vi "Read from Hardware.vi"(8 "error in":errorcluster, 10 "Values in":dbl[](array[numeric]), 11 "Tx Execution Unit Implementation in":refnum<class "Tx Generic Execution Unit.lvclass">) -> (0 "error out":errorcluster, 2 "Values out":dbl[](array[numeric]), 3 "Tx Execution Unit Implementation out":refnum<class "Tx Generic Execution Unit.lvclass">)   [LabVIEW 2025, in "AIM ARINC 664 Engine.lvlib" / "Implementation.lvlib" / "Tx Generic Execution Unit.lvclass"]
uses:
  Tx Generic Execution Unit.lvclass
  Tx Generic Execution Unit.lvclass/Tx Generic Execution Unit.ctl
  <instrlib>/AIM GmbH/_AIM 664/AIM664LV.lvlib
  <vilib>/Utility/SystemLogging/NI_SystemLogging.lvlib
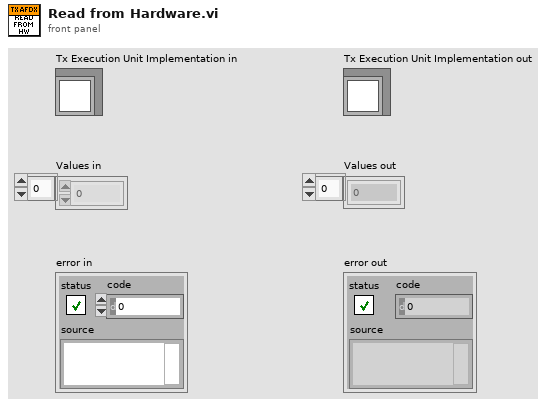
[diagram p1: front panel]
types:
  T1 = cluster{"QueueStatus":i32, "BytesReloadable":u32, "FramesSent":u32, "FramesInCycQueue":u32}
  T2 = cluster{"TxStatus":u32, "Frames":u32, "TransmitMode":u32, "FramesPortB":u32}
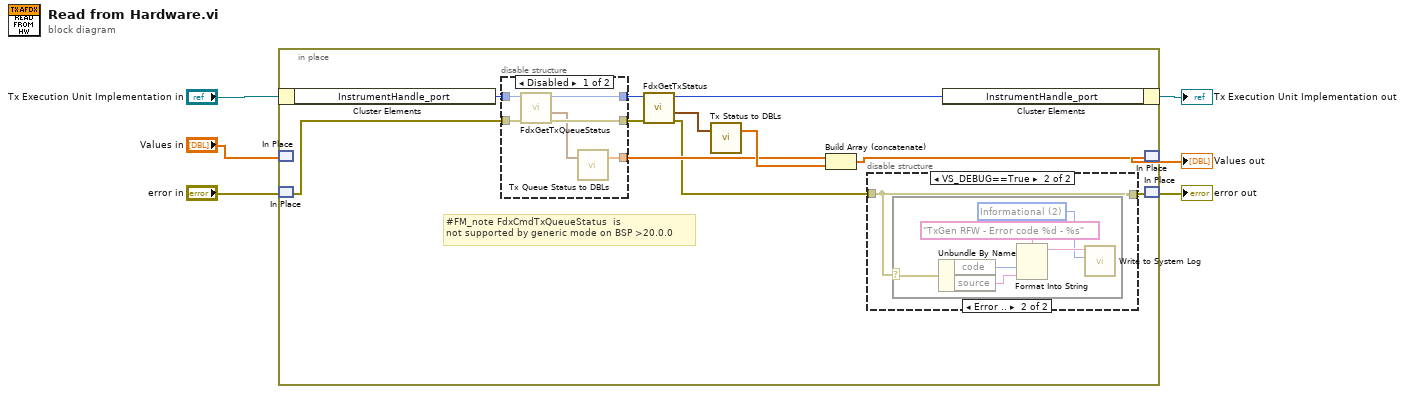
[diagram p0: block diagram]
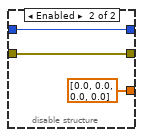
[diagram p2: hidden frame]
diagram:
  n1 = in-place {
    # "#FM_note FdxCmdTxQueueStatus  is \nnot supported by generic mode on BSP >20.0.0"
    n2 = in-place-cluster #1("Tx Execution Unit Implementation in") -> ("InstrumentHandle_port"=w16:u32)
    n3 = in-place-match #2("Values in") -> ()  [unwired: 1 out]
    n4 = in-place-match #3("error in") -> (w14:errorcluster)
    n5 = disable-structure shown="Disabled" {
      disable-tunnel: [w23 w26] -> w17
      disable-tunnel: w16 -> [w22 w25]
      disable-tunnel: [w21 w25] -> w15
      disable-tunnel: w14 -> [w20 w26]
      disable-tunnel: [w18 dbl[] [0.0, 0.0, 0.0, 0.0] ("TxQueueStatusDBLs")] -> w10
      frame Disabled {
        n6 = call <instrlib>:"FdxGetTxQueueStatus.vi"("error in"=w20, "InstrumentHandle"=w22) -> ("error out"=w23:errorcluster, "TxQueueStatus"=w19:T1, "InstrumentHandle"=w21:u32)  [unwired: 7 in]
        n7 = call "Tx Queue Status to DBLs.vi"("TxQueueStatus"=w19) -> ("TxQueueStatusDBLs"=w18:dbl[])  [unwired: 2 in]
      }
      frame Enabled {
      }
    }
    n8 = call <instrlib>:"FdxGetTxStatus.vi"("error in"=w17, "InstrumentHandle_port"=w15) -> ("error out"=w8:errorcluster, "TxStatus"=w12:T2, "InstrumentHandle_port"=w13:u32)  [unwired: 7 in]
    n9 = call "Tx Status to DBLs.vi"("TxStatus"=w12) -> ("TxStatusDBLs"=w11:dbl[])  [unwired: 2 in]
    n10 = Build Array (concatenate)(w10, w11) -> (w9:dbl[])
    n11 = disable-structure shown="VS_DEBUG==True" {
      disable-tunnel: w8 -> [w27 w28]
      disable-tunnel: [w27 w28] -> w7
      frame condition #0 (active) {
      }
      frame condition #1 {
        n12 = case shown="Error .." w28 {
          selector: w28 -> [_ w29]
          frame No Error {
          }
          frame Error {
            w32 = 2 items=["Error", "Warning", "Informational"] ("severity")
            n13 = Unbundle By Name(w29) -> ("code"=w31:i32, "source"=w30:string)
            n14 = Format Into String(format string="TxGen RFW - Error code %d - %s", w31, w30) -> (resulting string=w33:string)  [unwired: 2 in, 1 out]
            n15 = call <vilib>:"Write to System Log.vi"("severity"=w32, "message"=w33) -> ()  [unwired: 9 in, 1 out]
          }
        }
      }
    }
    n16 = in-place-cluster #1("InstrumentHandle_port"=w13) -> (→"Tx Execution Unit Implementation out":refnum<class "Tx Generic Execution Unit.lvclass">)
    n17 = in-place-match #2(w9) -> (→"Values out":dbl[])
    n18 = in-place-match #3(w7) -> (→"error out":errorcluster)
  }
